vi "Case_Statement.vi"() -> ()   [LabVIEW 2015]
uses:
  <vilib>/express/express arith-compare/Formula/XNode/ExpressFormulaBlockNode.xnode
panel:
  in  "input variable":dbl
  out "output variable":dbl
  in  "Boolean":bool
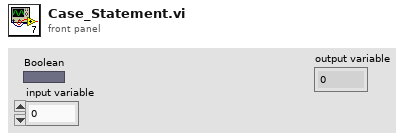
[diagram p1: front panel]
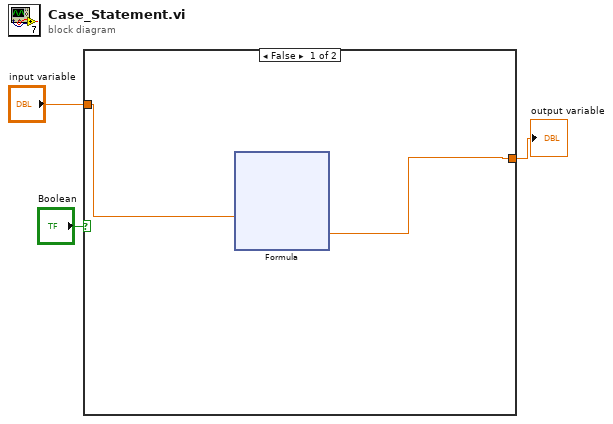
[diagram p0: block diagram]
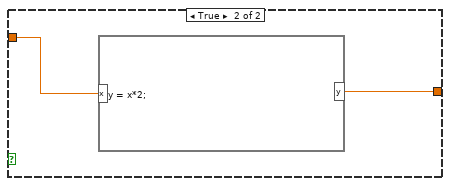
[diagram p2: hidden frame]
diagram:
  n1 = case shown="False" "Boolean" {
    tunnel: "input variable" -> [w5 w15]
    tunnel: [w4 w14] -> w2
    frame False {
      n2 = xnode "Formula"("x"=w5) -> ("Result"=w4:dbl)  [unwired: 1 in, 1 out]
    }
    frame True {
      n3 = formula code="y = x*2;"("x"=w15) -> ("y"=w14:dbl)
    }
  }
  "output variable" <- w2
